vi "Define.vi"(11 "Relation Definition":T1) -> (3 "Entity out":refnum<class "Entity.lvclass">)   [LabVIEW 2020, in "Conditu2.lvlib" / "Columns.lvlib" / "Entity.lvclass"]
uses:
  Entity.lvclass
  C:/dev/lv20CE/lv-conditum-tools/Conditum-Clone/Columns/Relation/Relation.lvclass
  Relation/Relation Definition.ctl
  Type/Definition.ctl
  Relation/Relation Info.ctl
  Relation Mapping.ctl
  Type/Type.lvclass/Type.ctl
  Relation/Relation.lvclass/Relation.ctl
  Type/Define Type.vi
  Relation/Relation.lvclass
  C:/dev/lv20CE/lv-conditum-tools/Conditum-Clone/Columns/Type/Type.lvclass
  Conditu2.lvlib
  Type/Type.lvclass
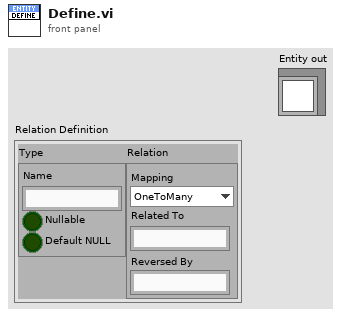
[diagram p1: front panel]
types:
  T1 = typedef "Conditu2.lvlib/Columns.lvlib/Relation.lvclass/Relation Definition.ctl" = cluster{"Type":T2, "Relation":T3}
  T2 = typedef "Conditu2.lvlib/Columns.lvlib/Type.lvclass/Definition.ctl" = cluster{"Name":string, "Nullable":bool, "Default NULL":bool}
  T3 = typedef "Conditu2.lvlib/Relation Info.ctl" = cluster{"Mapping":T4, "Related To":string, "Reversed By":string}
  T4 = typedef "Conditu2.lvlib/Relation Mapping.ctl" = enum16{"OneToMany", "ManyToOne", "ManyToMany", "OneToOne"}
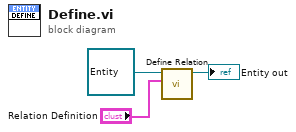
[diagram p0: block diagram]
diagram:
  n1 = call "Define Relation.vi"("Relation Definition"="Relation Definition", "Relation in"=refnum<class "Entity.lvclass"> refnum ("Entity out")) -> ("Relation out"=→"Entity out":refnum<class "Entity.lvclass">)  [unwired: 9 in]
